vi "DriveSet6(SubVI).vi"(9 "Left":dbl format="%#_13g", 10 "Right":dbl format="%#_13g", 11 "output cluster":T1) -> (3 "appended array":dbl[](array[numeric]))   [LabVIEW 2017]
uses:
  FRC SimulatedRSC/DriveMotors.ctl
  <vilib>/Rock Robotics/WPI/MotorControl/WPI_MotorControlDeviceRef.ctl
  <vilib>/Rock Robotics/WPI/MotorControl/WPI_MotorControlType.ctl
  <vilib>/Rock Robotics/SystemInterfaces/DIO/FPGA_DIOPWMChannel.ctl
  <vilib>/Rock Robotics/WPI/PWM/WPI_PWMDeadband.ctl
  <vilib>/Rock Robotics/SystemInterfaces/DIO/FPGA_DIOChannel.ctl
  Public/Documents/Cross The Road Electronics/Phoenix-LabVIEW/Motor Controller/Controls/CTRE_Phoenix_MotorControl_ControlMode.ctl
  Public/Documents/Cross The Road Electronics/Phoenix-LabVIEW/Motor Controller/Get/CTRE_Phoenix_MotorController_GetSelectedSensorData.vi
  <vilib>/Rock Robotics/Network Tables/NT Read Number.vi
panel:
  in  "PhaseSensor Left":bool
  in  "Invert Left":bool
  in  "PhaseSensor Right":bool
  in  "Invert Right":bool
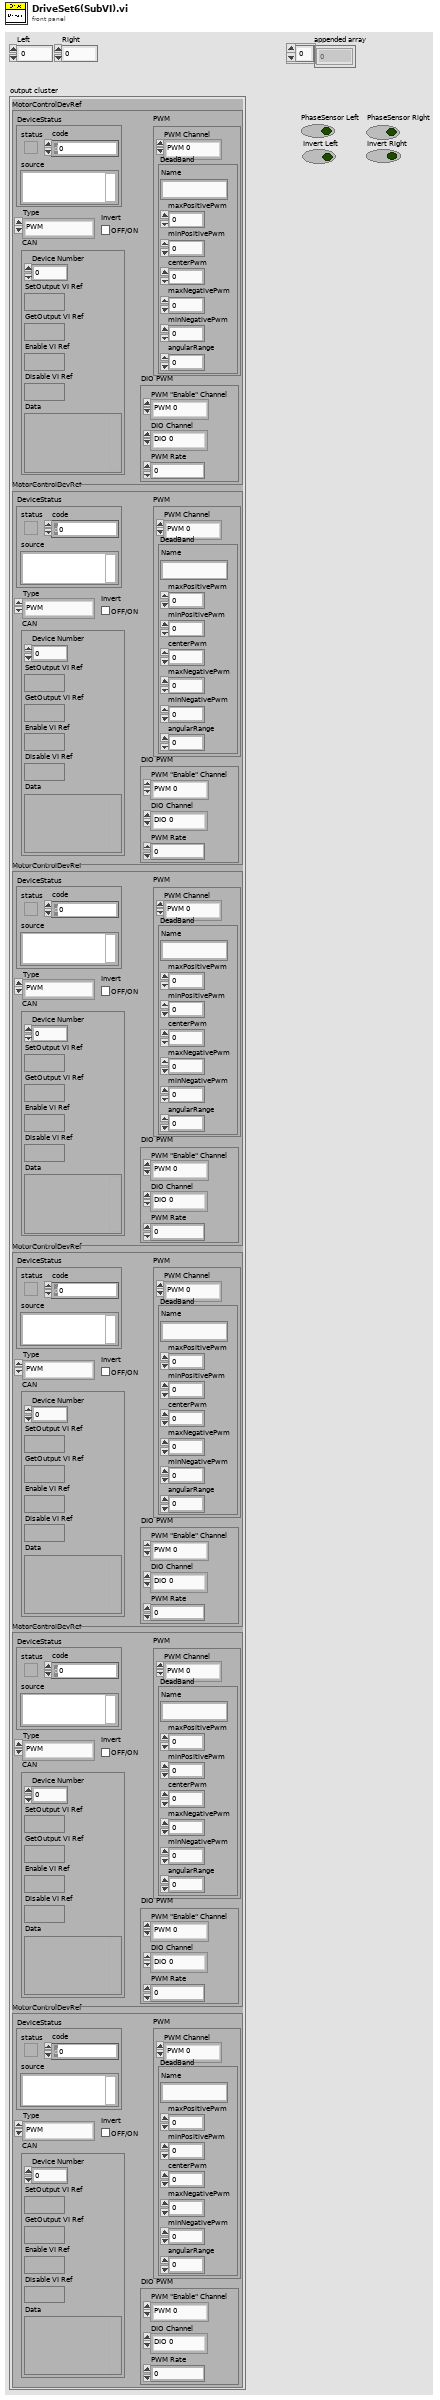
[diagram p1: front panel]
types:
  T1 = typedef "DriveMotors.ctl" = cluster{"MotorControlDevRef":T2, "MotorControlDevRef":T2, "MotorControlDevRef":T2, "MotorControlDevRef":T2, "MotorControlDevRef":T2, "MotorControlDevRef":T2}
  T2 = typedef "WPI_MotorControlDeviceRef.ctl" = cluster{"DeviceStatus":errorcluster, "Type":T3, "PWM":cluster{"PWM Channel":T4, "DeadBand":T5}, "CAN":cluster{"Device Number":u8, "SetOutput VI Ref":variant, "GetOutput VI Ref":variant, "Enable VI Ref":variant, "Disable VI Ref":variant, "Data":variant}, "Invert":bool, "DIO PWM":cluster{"PWM \"Enable\" Channel":T4, "DIOChannel":T6, "PWM Rate":dbl}}
  T3 = typedef "WPI_MotorControlType.ctl" = enum16{"PWM", "CAN", "DIO PWM"}
  T4 = typedef "FPGA_DIOPWMChannel.ctl" = enum8{"PWM 0", "PWM 1", "PWM 2", "PWM 3", "PWM 4", "PWM 5", "PWM 6", "PWM 7", "PWM 8", "PWM 9", "PWM MXP 0", "PWM MXP 1", "PWM MXP 2", "PWM MXP 3", "PWM MXP 4", "PWM MXP 5", "PWM MXP 6", "PWM MXP 7", "PWM MXP 8", "PWM MXP 9", "Invalid"}
  T5 = typedef "WPI_PWMDeadband.ctl" = cluster{"Name":string, "maxPositivePwm":i32, "minPositivePwm":i32, "centerPwm":i32, "maxNegativePwm":i32, "minNegativePwm":i32, "angularRange":u16}
  T6 = typedef "FPGA_DIOChannel.ctl" = enum8{"DIO 0", "DIO 1", "DIO 2", "DIO 3", "DIO 4", "DIO 5", "DIO 6", "DIO 7", "DIO 8", "DIO 9", "DIO MXP 0", "DIO MXP 1", "DIO MXP 2", "DIO MXP 3", "DIO MXP 4", "DIO MXP 5", "DIO MXP 6", "DIO MXP 7", "DIO MXP 8", "DIO MXP 9", "DIO MXP 10", "DIO MXP 11", "DIO MXP 12", "DIO MXP 13", "DIO MXP 14", "DIO MXP 15", "SPI Port CS1", "SPI Port CS2", "SPI Port CS3", "SPI Port MISO", "SPI Port MOSI", "Invalid"}
  T7 = typedef "CTRE_Phoenix_MotorControl_ControlMode.ctl" = u16
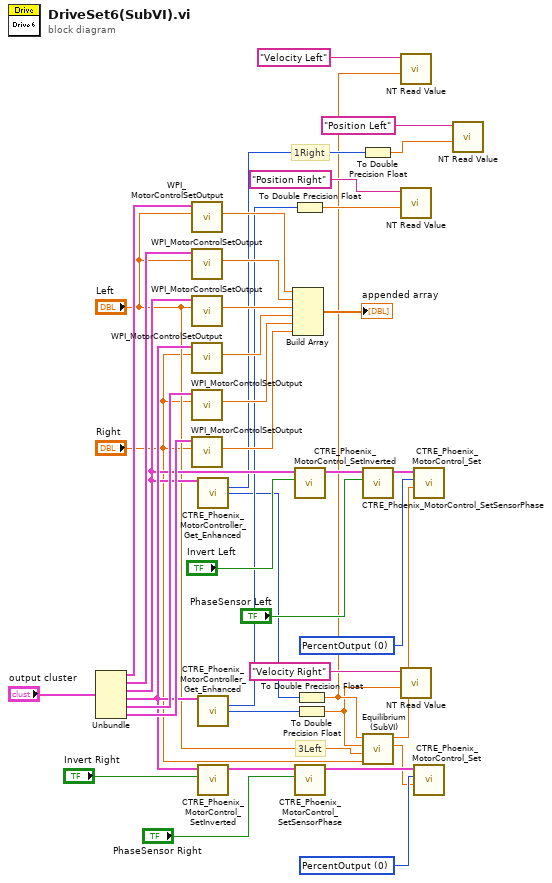
[diagram p0: block diagram]
diagram:
  w19 = T7 0 items=["PercentOutput"=0, "Position"=1, "Velocity"=2, "Current"=3, "Follower"=5, "MotionProfile"=6, "MotionMagic"=7, "MotionMagicArc"=8, "MotionProfileArc"=10, "Disabled"=15] ("Control Mode")
  w24 = T7 0 items=["PercentOutput"=0, "Position"=1, "Velocity"=2, "Current"=3, "Follower"=5, "MotionProfile"=6, "MotionMagic"=7, "MotionMagicArc"=8, "MotionProfileArc"=10, "Disabled"=15] ("Control Mode")
  # "3Left"
  # "1Right"
  n1 = Unbundle("output cluster") -> ("MotorControlDevRef"=w40:T2, "MotorControlDevRef"=w39:T2, "MotorControlDevRef"=w17:T2, "MotorControlDevRef"=w18:T2, "MotorControlDevRef"=w37:T2, "MotorControlDevRef"=w36:T2)
  n2 = call <vilib>:"WPI_MotorControlSetOutput.vi"("Output"="Left", "MotorControlDevRef"=w40) -> ("Motor Output"=w35:dbl)  [unwired: 7 in, 2 out]
  n3 = call <vilib>:"WPI_MotorControlSetOutput.vi"("Output"="Left", "MotorControlDevRef"=w39) -> ("Motor Output"=w34:dbl)  [unwired: 7 in, 2 out]
  n4 = call <vilib>:"WPI_MotorControlSetOutput.vi"("Output"="Left", "MotorControlDevRef"=w17) -> ("Motor Output"=w33:dbl)  [unwired: 7 in, 2 out]
  n5 = call <vilib>:"WPI_MotorControlSetOutput.vi"("Output"="Right", "MotorControlDevRef"=w18) -> ("Motor Output"=w32:dbl)  [unwired: 7 in, 2 out]
  n6 = call <vilib>:"WPI_MotorControlSetOutput.vi"("Output"="Right", "MotorControlDevRef"=w37) -> ("Motor Output"=w31:dbl)  [unwired: 7 in, 2 out]
  n7 = call <vilib>:"WPI_MotorControlSetOutput.vi"("Output"="Right", "MotorControlDevRef"=w36) -> ("Motor Output"=w30:dbl)  [unwired: 7 in, 2 out]
  n8 = call-poly "CTRE_Phoenix_MotorController_Get_Enhanced.vi"("PhoenixMotorControlDevRef"=w17) -> ("Position (Raw Sensor Units)"=w13:i32, "Velocity (Raw Sensor Units per 100 ms)"=w1:i32)  [unwired: 11 in, 2 out]
  n9 = call-poly "CTRE_Phoenix_MotorController_Get_Enhanced.vi"("PhoenixMotorControlDevRef"=w18) -> ("Position (Raw Sensor Units)"=w16:i32, "Velocity (Raw Sensor Units per 100 ms)"=w2:i32)  [unwired: 11 in, 2 out]
  n10 = call "CTRE_Phoenix_MotorControl_SetInverted.vi"("Invert?"="Invert Right", "PhoenixMotorControlDevRef"=w18) -> ("PhoenixMotorControlDevRef"=w28:T2)  [unwired: 8 in, 1 out]
  n11 = Build Array(w35, w34, w33, w32, w31, w30) -> (→"appended array":dbl[])
  n12 = To Double Precision Float(number=w16) -> (double precision float=w9:dbl)
  n13 = call "CTRE_Phoenix_MotorControl_SetInverted.vi"("Invert?"="Invert Left", "PhoenixMotorControlDevRef"=w17) -> ("PhoenixMotorControlDevRef"=w23:T2)  [unwired: 8 in, 1 out]
  n14 = call "CTRE_Phoenix_MotorControl_SetSensorPhase.vi"("PhaseSensor"="PhaseSensor Right", "PhoenixMotorControlDevRef"=w28) -> ("PhoenixMotorControlDevRef"=w27:T2)  [unwired: 8 in, 1 out]
  n15 = To Double Precision Float(number=w1) -> (double precision float=w8:dbl)
  n16 = To Double Precision Float(number=w2) -> (double precision float=w7:dbl)
  n17 = To Double Precision Float(number=w13) -> (double precision float=w10:dbl)
  n18 = call "CTRE_Phoenix_MotorControl_SetSensorPhase.vi"("PhaseSensor"="PhaseSensor Left", "PhoenixMotorControlDevRef"=w23) -> ("PhoenixMotorControlDevRef"=w22:T2)  [unwired: 8 in, 1 out]
  n19 = call "Equilibrium (SubVI).vi"("Right"=w8, "Left"=w7, "Left Output"="Left", "Right Output"="Right") -> ("Left Output New"=w4:dbl, "Right Output New"=w3:dbl)  [unwired: 5 in]
  n20 = call-poly <vilib>:"NT Read Value.vi"("Default Value"=w8, "Name"="Velocity Left") -> ()  [unwired: 8 in, 2 out]
  n21 = call-poly <vilib>:"NT Read Value.vi"("Default Value"=w9, "Name"="Position Right") -> ()  [unwired: 8 in, 2 out]
  n22 = call-poly <vilib>:"NT Read Value.vi"("Default Value"=w7, "Name"="Velocity Right") -> ()  [unwired: 8 in, 2 out]
  n23 = call "CTRE_Phoenix_MotorControl_Set.vi"("Output"=w4, "Control Mode"=w19, "PhoenixMotorControlDevRef"=w22) -> ()  [unwired: 7 in, 2 out]
  n24 = call "CTRE_Phoenix_MotorControl_Set.vi"("Output"=w3, "Control Mode"=w24, "PhoenixMotorControlDevRef"=w27) -> ()  [unwired: 7 in, 2 out]
  n25 = call-poly <vilib>:"NT Read Value.vi"("Default Value"=w10, "Name"="Position Left") -> ()  [unwired: 8 in, 2 out]
